vi "TS FIFOs5 ch 1 sample resonance scanner (FPGA) fixed pix clock.vi"() -> ()   [LabVIEW 2012]
uses:
  <vilib>/eio/EIONode/EIONode.xnode
  <vilib>/rvi/eio/common/nirviEmuTemplateMethod_errors.vi
  <vilib>/Platform/TimedLoop/XDataNode/XDataNode.xnode
  <vilib>/Platform/TimedLoop/XDataNode/nitl_modes.ctl
  <vilib>/Platform/TimedLoop/XDataNode/XDNodeRunTimeDep.lvlib
  <vilib>/Platform/TimedLoop/XDataNode/wakeup.ctl
  <vilib>/Platform/TimedLoop/XDataNode/timing_clust.ctl
  <vilib>/rvi/DataTransferAndStorage/Container/XNode/niFpgaContainer.xnode
  <vilib>/rvi/FIFO/Fifo_Resource/nirvififoEmulationWrite.vi
  <vilib>/rvi/FIFO/Fifo_Resource/nirvififoEmulationRead.vi
  <vilib>/rvi/interface/RandomDataEmulation/nirviRandomDataFpgaReadWriteTemplate.vi
panel:
  in  "lines at once":i16=4999
  in  "samples per half period":i16=4999
  in  "Start Delay (Ticks)":i16 caption="Start delay (Ticks)"
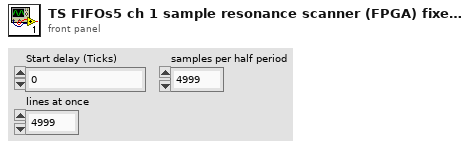
[diagram p1: front panel]
types:
  T1 = typedef "XDNodeRunTimeDep.lvlib/timing_clust.ctl" = cluster{"Expected End [f-1]":u64, "Actual End [f-1]":u64, "Finished Late? [f-1]":bool, "Expected End [i-1]":u64, "Actual End [i-1]":u64, "Finished Late? [i-1]":bool, "Expected Start [i]":u64, "Actual Start [i]":u64, "Expected Start [f]":u64, "Actual Start [f]":u64, "Source Name":string, "Structure Name":string, "Period":i64, "Deadline":i64, "Offset":i64, "Start":i64, "Priority":i32, "Timeout":i32, "Mode":T2, "Wakeup Reason":T3, "Error":errorcluster, "Source Type":string, "Secondary Source Type":string, "Global End Time":u64, "Global Start Time":u64, "Frame Duration":u64, "Iteration Duration":u64, "Assigned CPU":i32, "I/O Scan Engine Mode":u32}
  T2 = typedef "XDNodeRunTimeDep.lvlib/nitl_modes.ctl" = enum32{"No Change", "Process missed periods, maintain original phase", "Discard missed periods, maintain original phase", "Process missed periods, ignore original phase", "Discard missed periods, ignore original phase"}
  T3 = typedef "XDNodeRunTimeDep.lvlib/wakeup.ctl" = enum32{"Normal", "Aborted", "Asynchronous wakeup", "Timing source error", "Timed loop error", "Timeout"}
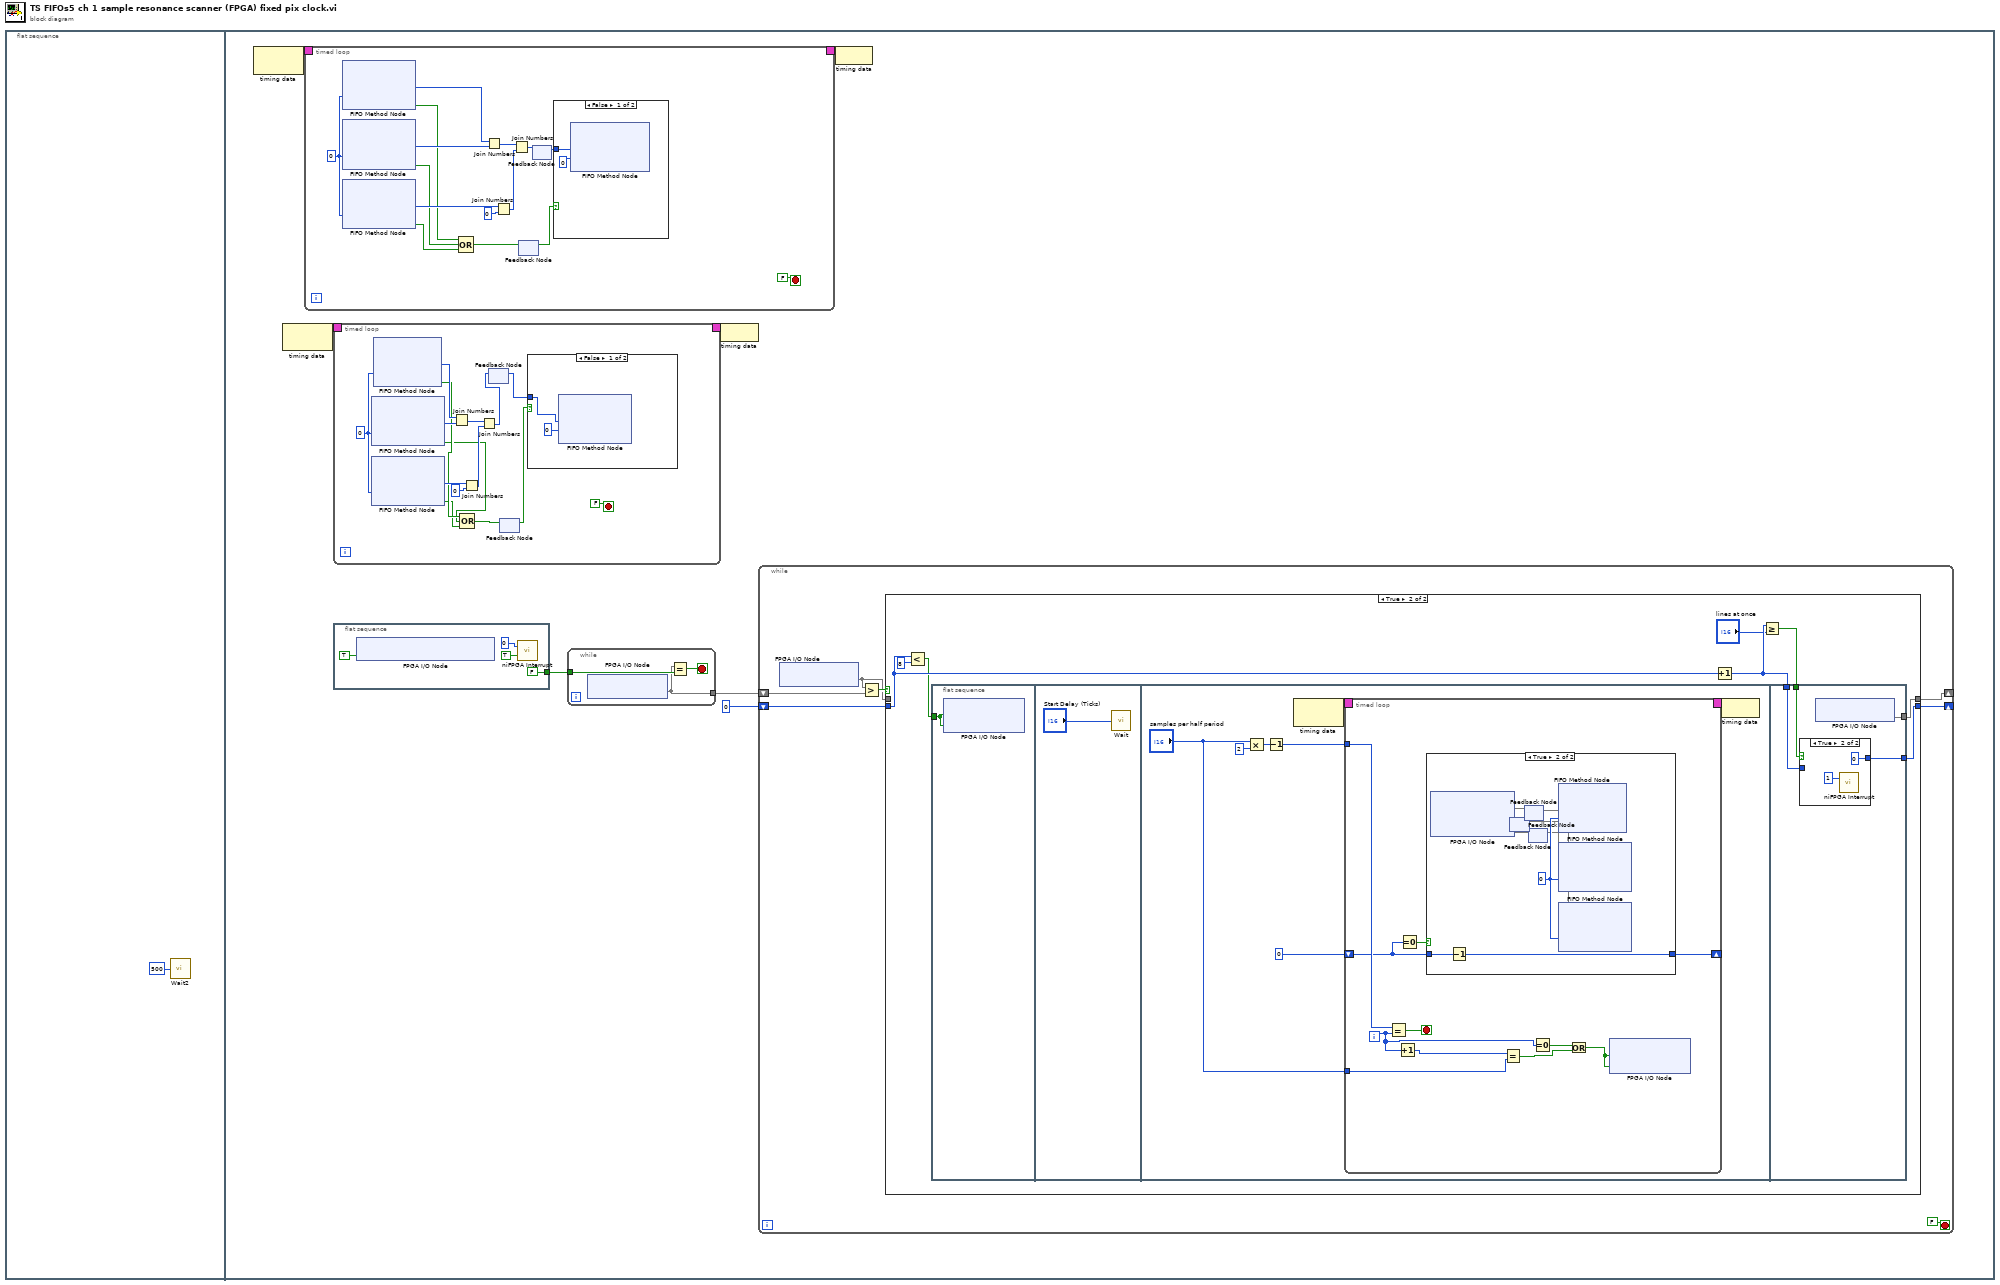
[diagram p0: block diagram]
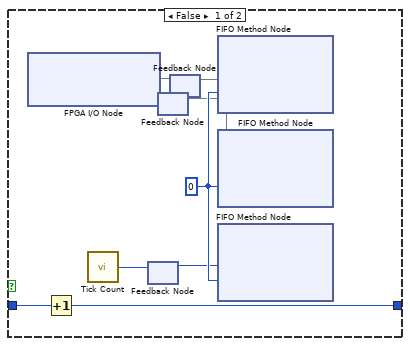
[diagram p5: hidden frame]
diagram:
  n1 = flat-sequence {
    frame #0 {
      n2 = call "Wait2"("Count(mSec)"=u32 500) -> ()  [unwired: 1 out]
    }
    frame #1 {
      n3 = node-c288() -> (w6:T1)  [unwired: 1 in]
      n4 = node-c288() -> (w8:T1)  [unwired: 1 in]
      n5 = timed-loop {
        timing: w6 -> [_]
        timing-out: [_] -> w5
        stop <- FALSE stop-if-true
        w23 = 0 ("Timeout")
        n6 = xnode ("FIFO Method Node")("Timeout"=w23) -> ("Element"=w19:i16, "Timed Out?"=w13:bool)  [unwired: 1 in, 1 out]
        n7 = xnode ("FIFO Method Node")("Timeout"=w23) -> ("Element"=w18:i16, "Timed Out?"=w12:bool)  [unwired: 1 in, 1 out]
        n8 = xnode ("FIFO Method Node")("Timeout"=w23) -> ("Element"=w17:i16, "Timed Out?"=w11:bool)  [unwired: 1 in, 1 out]
        n9 = Compound Arithmetic op=OR(w13, w12, w11) -> (w10:bool)
        n10 = Join Numbers(hi=w19, lo=w18) -> ((hi.lo)=w21:u32)
        n11 = Join Numbers(hi=w17, lo=i16 0) -> ((hi.lo)=w20:u32)
        n12 = Join Numbers(hi=w21, lo=w20) -> ((hi.lo)=w22:u64)
        n13 = feedback-in #1(w10) -> ()
        n14 = feedback #1() -> (w9:bool)  [unwired: 1 in]
        n15 = feedback-in #2(w22) -> ()
        n16 = feedback #2() -> (w14:u64)  [unwired: 1 in]
        n17 = case shown="False" w9 {
          tunnel: w14 -> [w24 _]
          frame False {
            n18 = xnode ("FIFO Method Node")("Element"=w24, "Timeout"=0) -> ()  [unwired: 1 in, 2 out]
          }
          frame True {
          }
        }
      }
      n19 = timed-loop {
        timing: w8 -> [_]
        timing-out: [_] -> w7
        stop <- FALSE stop-if-true
        w39 = 0 ("Timeout")
        n20 = xnode ("FIFO Method Node")("Timeout"=w39) -> ("Element"=w41:i16, "Timed Out?"=w32:bool)  [unwired: 1 in, 1 out]
        n21 = xnode ("FIFO Method Node")("Timeout"=w39) -> ("Element"=w40:i16, "Timed Out?"=w31:bool)  [unwired: 1 in, 1 out]
        n22 = xnode ("FIFO Method Node")("Timeout"=w39) -> ("Element"=w42:i16, "Timed Out?"=w33:bool)  [unwired: 1 in, 1 out]
        n23 = Join Numbers(hi=w42, lo=w41) -> ((hi.lo)=w43:u32)
        n24 = Compound Arithmetic op=OR(w33, w32, w31) -> (w34:bool)
        n25 = Join Numbers(hi=w40, lo=i16 0) -> ((hi.lo)=w44:u32)
        n26 = Join Numbers(hi=w43, lo=w44) -> ((hi.lo)=w36:u64)
        n27 = feedback #3() -> (w35:u64)  [unwired: 1 in]
        n28 = feedback-in #3(w36) -> ()
        n29 = feedback #4() -> (w30:bool)  [unwired: 1 in]
        n30 = feedback-in #4(w34) -> ()
        n31 = case shown="False" w30 {
          tunnel: w35 -> [w45 _]
          frame False {
            n32 = xnode ("FIFO Method Node")("Element"=w45, "Timeout"=0) -> ()  [unwired: 1 in, 2 out]
          }
          frame True {
          }
        }
      }
      n33 = flat-sequence {
        tunnel: [FALSE ("IO Module\\DI 0")] -> w3
        frame #0 {
          n34 = xnode "FPGA I/O Node"("IO Module\\Digital Output Enable"=TRUE ("IO Module\\Digital Output Enable")) -> ()  [unwired: 1 in, 1 out]
          n35 = call <vilib>:"niFPGA Interrupt.vi"("Wait Until Cleared (F)"=TRUE, "IRQ Number (0)"=u8 0) -> ()  [unwired: 1 in]
        }
      }
      n36 = while {
        tunnel: w3 -> [w53]
        tunnel: [w51] -> w2
        stop <- w52 stop-if-true
        n37 = xnode "FPGA I/O Node"() -> ("IO Module\\DI 0"=w51)  [unwired: 1 in, 1 out]
        n38 = Equal?(x=w51, y=w53) -> (x = y?=w52:bool)
      }
      n39 = node-c288(w7) -> ()
      n40 = while {
        shift-right: [w63] -> _
        shift-left: w2 -> [w64]
        shift-right: [w61] -> _
        shift-left: i16 0 ("IRQ Number (0)") -> [w60]
        stop <- FALSE stop-if-true
        n41 = xnode "FPGA I/O Node"() -> ("IO Module\\DI 0"=w58)  [unwired: 1 in, 1 out]
        n42 = Greater?(x=w58, y=w64) -> (0:w59:bool)
        n43 = case shown="True" w59 {
          tunnel: [w65 w67] -> w63
          tunnel: w60 -> [w66 w70]
          tunnel: [w66 w72] -> w61
          tunnel: w58 -> [w65 _]
          frame False {
          }
          frame True {
            n44 = Less?(x=w70, y=i16 8) -> (x < y?=w68:bool)
            n45 = flat-sequence {
              tunnel: w68 -> [w75]
              tunnel: w74 -> [w120]
              tunnel: w73 -> [w119]
              tunnel: [w118] -> w72
              tunnel: [w117] -> w67
              frame #0 {
                n46 = xnode "FPGA I/O Node"("PXI_Trig2"=w75, "IO Module\\D0 2"=w75) -> ()  [unwired: 2 in, 2 out]
              }
              frame #1 {
                n47 = call "Wait"("Count(Ticks)"="Start Delay (Ticks)") -> ()  [unwired: 1 out]
              }
              frame #2 {
                n48 = Multiply(x="samples per half period", y=i16 2) -> (x*y=w82:i16)
                n49 = Decrement(x=w82) -> (x-1=w78:i16)
                n50 = node-c288() -> (w81:T1)  [unwired: 1 in]
                n51 = timed-loop {
                  tunnel: w78 -> [w93]
                  timing: w81 -> [_]
                  timing-out: [_] -> w80
                  shift-right: [w90] -> _
                  shift-left: 0 ("Timeout") -> [w91]
                  tunnel: "samples per half period" -> [w85]
                  i -> [w84]
                  stop <- w94 stop-if-true
                  n52 = Equal?(x=w93, y=w84) -> (x = y?=w94:bool)
                  n53 = Increment(x=w84) -> (x+1=w86:i32)
                  n54 = Equal To 0?(x=w91) -> (x = 0?=w92:bool)
                  n55 = case shown="True" w92 {
                    tunnel: w91 -> [w103 w112]
                    tunnel: [w102 w111] -> w90
                    frame False {
                      w101 = 0 ("Timeout")
                      n56 = xnode "FPGA I/O Node"() -> ("IO Module\\AI A6"=w100, "IO Module\\AI B8"=w99)  [unwired: 2 in, 2 out]
                      n57 = Increment(x=w103) -> (x+1=w102:i32)
                      n58 = call "Tick Count"() -> ("Tick Count(Ticks)"=w98:u32)
                      n59 = feedback-in #5(w98) -> ()
                      n60 = feedback #5() -> (w97:u32)  [unwired: 1 in]
                      n61 = feedback-in #6(w99) -> ()
                      n62 = feedback #6() -> (w96)  [unwired: 1 in]
                      n63 = feedback-in #7(w100) -> ()
                      n64 = feedback #7() -> (w95)  [unwired: 1 in]
                      n65 = xnode ("FIFO Method Node")("Element"=w95, "Timeout"=w101) -> ()  [unwired: 1 in, 2 out]
                      n66 = xnode ("FIFO Method Node")("Element"=w96, "Timeout"=w101) -> ()  [unwired: 1 in, 2 out]
                      n67 = xnode ("FIFO Method Node")("Element"=w97, "Timeout"=w101) -> ()  [unwired: 1 in, 2 out]
                    }
                    frame True {
                      w107 = 0 ("Timeout")
                      n68 = xnode "FPGA I/O Node"() -> ("IO Module\\AI A0"=w110, "IO Module\\AI A1"=w109, "IO Module\\AI A3"=w108)  [unwired: 3 in, 3 out]
                      n69 = Decrement(x=w112) -> (x-1=w111:i32)
                      n70 = feedback-in #8(w109) -> ()
                      n71 = feedback #8() -> (w105)  [unwired: 1 in]
                      n72 = feedback-in #9(w110) -> ()
                      n73 = feedback #9() -> (w106)  [unwired: 1 in]
                      n74 = feedback-in #10(w108) -> ()
                      n75 = feedback #10() -> (w104)  [unwired: 1 in]
                      n76 = xnode ("FIFO Method Node")("Element"=w106, "Timeout"=w107) -> ()  [unwired: 1 in, 2 out]
                      n77 = xnode ("FIFO Method Node")("Element"=w105, "Timeout"=w107) -> ()  [unwired: 1 in, 2 out]
                      n78 = xnode ("FIFO Method Node")("Element"=w104, "Timeout"=w107) -> ()  [unwired: 1 in, 2 out]
                    }
                  }
                  n79 = Equal?(x=w86, y=w85) -> (x = y?=w88:bool)
                  n80 = Equal To 0?(x=w84) -> (x = 0?=w89:bool)
                  n81 = Or(x=w89, y=w88) -> (x .or. y?=w87:bool)
                  n82 = xnode "FPGA I/O Node"("IO Module\\D0 1"=w87, "PXI_Trig1"=w87) -> ()  [unwired: 2 in, 2 out]
                }
                n83 = node-c288(w80) -> ()
              }
              frame #3 {
                n84 = case shown="True" w119 {
                  tunnel: w120 -> [w121 _]
                  tunnel: [w121 u8 0] -> w118
                  frame False {
                  }
                  frame True {
                    n85 = call <vilib>:"niFPGA Interrupt.vi"("IRQ Number (0)"=u8 1) -> ()  [unwired: 2 in]
                  }
                }
                n86 = xnode "FPGA I/O Node"() -> ("IO Module\\DI 0"=w117)  [unwired: 1 in, 1 out]
              }
            }
            n87 = Increment(x=w70) -> (x+1=w74:i16)
            n88 = Greater Or Equal?(x=w74, y="lines at once") -> (x >= y?=w73:bool)
          }
        }
      }
      n89 = node-c288(w5) -> ()
    }
  }
